vi "udp_subscribe.vi"(8 "error in":errorcluster, 11 "UDP Subscriber":T2={"Update Period\n[.001 secs]"=50, "error out"={"status"=FALSE, "code"=0, "source"=""}, "Stop"=FALSE, "Activity"=FALSE, "Finished\nLate?"=FALSE, "Data Received"="", "UDP Configuration"={"connection ID"=refnum, "Local"={"Port "=60015, "Timeout (ms)"=30, "Max Packet Bytes"=1024}, "byte order"=enum."big-endian, network order", "incl. arr/str. size"=FALSE}, "data source info"={"address"="0.0.0.0", "port"=0}}) -> (0 "error out":errorcluster, 2 "Updating Data...":bool, 3 "UDP Subscriber (out)":T2={"Update Period\n[.001 secs]"=50, "error out"={"status"=FALSE, "code"=0, "source"=""}, "Stop"=FALSE, "Activity"=FALSE, "Finished\nLate?"=FALSE, "Data Received"="", "UDP Configuration"={"connection ID"=refnum, "Local"={"Port "=60015, "Timeout (ms)"=30, "Max Packet Bytes"=1024}, "byte order"=enum."big-endian, network order", "incl. arr/str. size"=FALSE}, "data source info"={"address"="0.0.0.0", "port"=0}}, 4 "Validated":bool, 6 "New Data Received":bool)   [LabVIEW 2014]
uses:
  typedefs/udp_subscriber.ctl
  typedefs/udp__sub_configuration.ctl
panel:
  in  "Tab Control":enum32{"Main", "I/O"}(tab)
  out "data out":string
  out "UDP Configuration":T1={"connection ID"=refnum, "Local"={"Port "=60015, "Timeout (ms)"=30, "Max Packet Bytes"=1024}, "byte order"=enum."big-endian, network order", "incl. arr/str. size"=FALSE}
  in  "IgnoreIP":string[](array[string])=["192.168.1.11", "0.0.0.0", "127.0.0.1", "0.0.0.6"]
  # "UDP Subscribe"
  # "UDP Subscribe:"
  # "UDP Subscribe:"
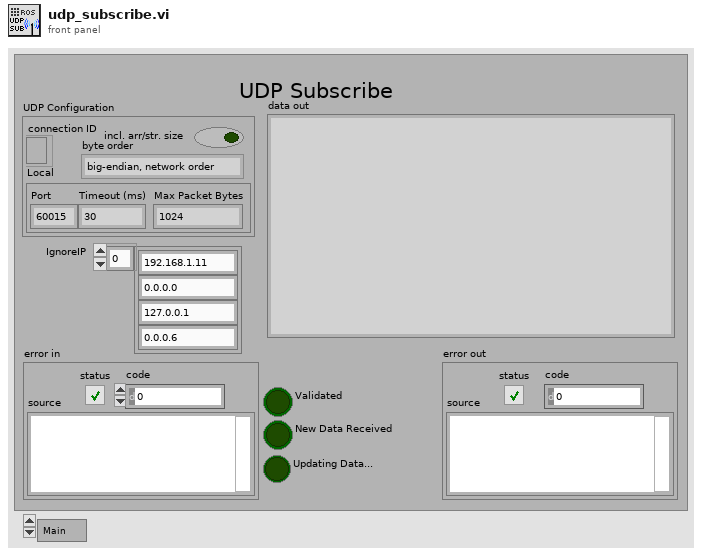
[diagram p1: front panel]
types:
  T1 = typedef "udp__sub_configuration.ctl" = cluster{"connection ID":refnum<k16>, "Local":cluster{"Port ":u16, "Timeout (ms)":i32, "Max Packet Bytes":i32}, "byte order":enum16{"big-endian, network order", "native, host order", "little-endian"}, "incl. arr/str. size":bool}
  T2 = typedef "udp_subscriber.ctl" = cluster{"Update Period\n[.001 secs]":i64, "error out":errorcluster, "Stop":bool, "Activity":bool, "Finished\nLate?":bool, "Data Received":string, "UDP Configuration":T1, "data source info":cluster{"address":string, "port":u16}}
  T3 = enum16{"big-endian, network order", "native, host order", "little-endian"}
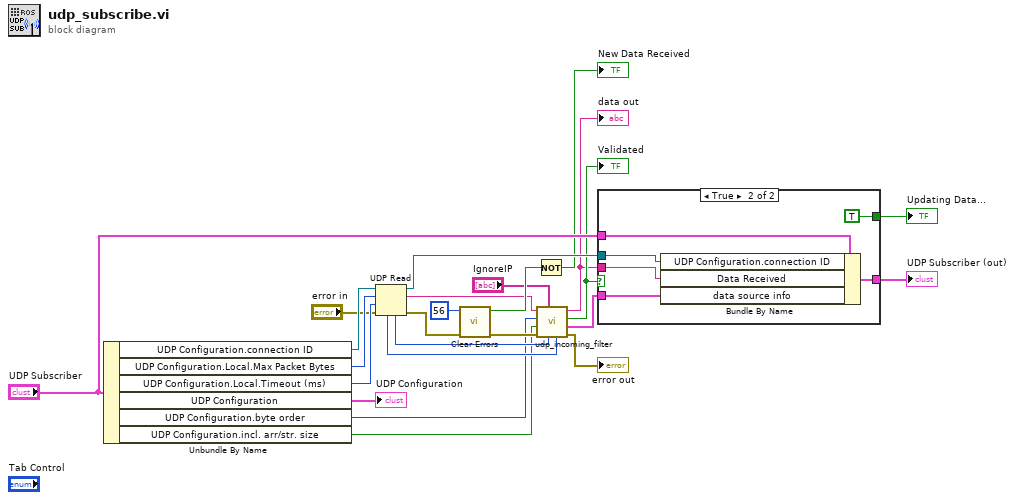
[diagram p0: block diagram]
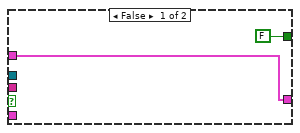
[diagram p2: hidden frame]
diagram:
  n1 = Unbundle By Name("UDP Subscriber") -> ("UDP Configuration.connection ID"=w22:refnum<k16>, "UDP Configuration.Local.Max Packet Bytes"=w23:i32, "UDP Configuration.Local.Timeout (ms)"=w24:i32, "UDP Configuration"=→"UDP Configuration":T1, "UDP Configuration.byte order"=w3:T3, "UDP Configuration.incl. arr/str. size"=w2:bool)
  n2 = UDP Read(connection ID=w22, max size (548)=w23, timeout ms (25000)=w24, 8:"error in") -> (data out=w4:string, error out=w18:errorcluster, 3:w14:refnum<k16>, 4:w10:u16, 6:w11:u32)
  n3 = call <vilib>:"Clear Errors.vi"("error in (no error)"=w18, "specific error code to clear (0: all)"=56) -> ("error out"=w9:errorcluster, "specific error cleared?"=w17:bool)  [unwired: 4 in]
  n4 = Not(x=w17) -> (.not. x?=→"New Data Received":bool)
  n5 = call "udp_incoming_filter.vi"("net address"=w11, "port"=w10, "IgnoreIP"="IgnoreIP", "error in (no error)"=w9, "data includes array or string size?"=w2, "byte order (0:big-endian, network order)"=w3, "received string"=w4) -> ("error out"=→"error out":errorcluster, "data source info"=w7:cluster{"name":string, "port":u16}, "Validated"=w6:bool, "data string"=w5:string)  [unwired: 1 in]
  "data out" <- w5
  "Validated" <- w6
  n6 = case shown="True" w6 {
    tunnel: [w26 w32] -> w16
    tunnel: "UDP Subscriber" -> [w26 w30]
    tunnel: w14 -> [_ w31]
    tunnel: w5 -> [_ w29]
    tunnel: w7 -> [_ w27]
    tunnel: [FALSE TRUE] -> w13
    frame False {
    }
    frame True {
      n7 = Bundle By Name(cluster=w30, "UDP Configuration.connection ID"=w31, "Data Received"=w29, "data source info"=w27) -> (w32:T2)
    }
  }
  "UDP Subscriber (out)" <- w16
  "Updating Data..." <- w13
